vi "Simple Solenoid.vi"() -> ()   [LabVIEW 2025]
doc: "Simple Solenoid Example\n\nThis example shows how to set the value of a Solenoid Channel.\n\nIt works with the PCM (Pneumatic Control Module) communicating with the roboRIO over CAN bus. The PCM must also be supplied with 12V DC from the PDP (Power Distribution Panel).\n\nThe Compressor, Pressure Switch, and Solenoid are all wired to the PCM \n\nThis example expects a USB cable connected from your development PC to the Type B USB Jack (next to the power input) on the roboRIO.\n\nThis example expects the Driver Station to be running."
uses:
  <vilib>/Rock Robotics/WPI/Solenoid/WPI_SolenoidChannel.ctl
  <vilib>/Rock Robotics/WPI/Solenoid/WPI_SolenoidValue.ctl
  <vilib>/Rock Robotics/WPI/Solenoid/WPI_SolenoidOpenSingle.vi
  <vilib>/Rock Robotics/WPI/Solenoid/WPI_SolenoidSetEnum.vi
panel:
  in  "Select a PD device by clicking on the image below":u16(ring) items=["CTRE Pneumatic Module", "REV Pneumatics Hub"]
  in  "Solenoid Channel":T1
  in  "Value to Write":bool
  in  "stop":bool
  # "Wiring Diagram"
  # "Set this input before running."
  # "This can be set while running."
  # "On"
  # "Off"
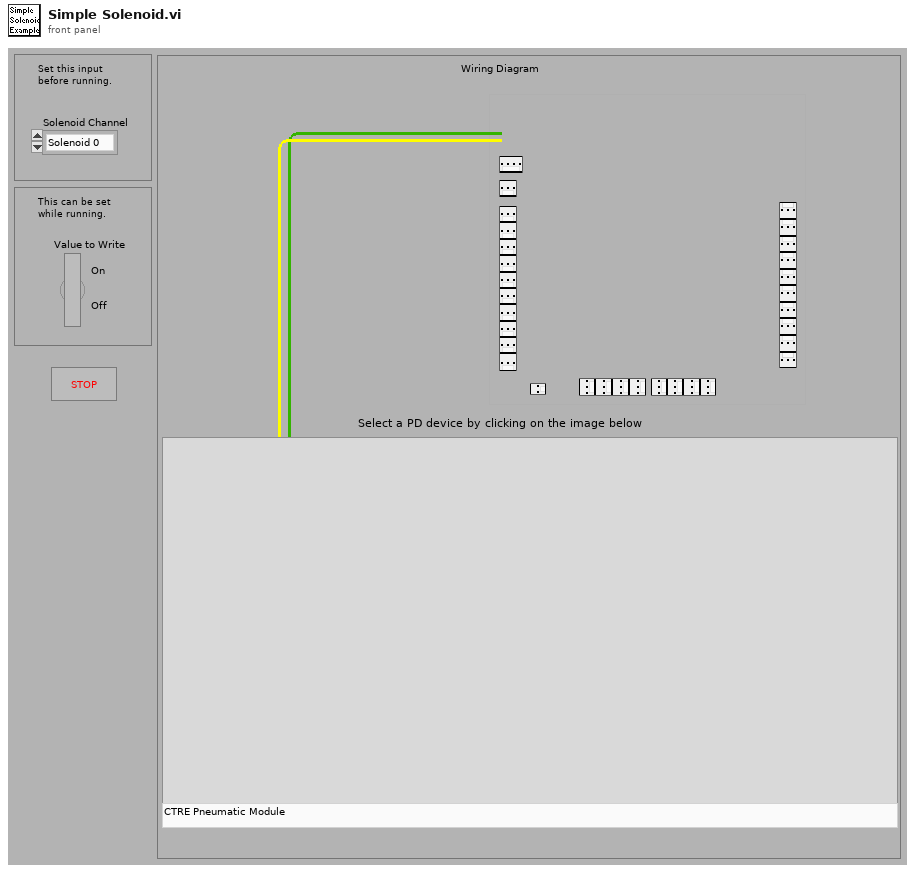
[diagram p1: front panel]
types:
  T1 = typedef "WPI_SolenoidChannel.ctl" = enum8{"Solenoid 0", "Solenoid 1", "Solenoid 2", "Solenoid 3", "Solenoid 4", "Solenoid 5", "Solenoid 6", "Solenoid 7", "Solenoid 8", "Solenoid 9", "Solenoid 10", "Solenoid 11", "Solenoid 12", "Solenoid 13", "Solenoid 14", "Solenoid 15", "Invalid"}
  T2 = typedef "WPI_SolenoidDevRef.ctl" = cluster{"DevStatus":errorcluster, "Pneumatics Control Module":u8, "Forward Solenoid Channel":T1, "Reverse Solenoid Channel":T1}
  T3 = typedef "WPI_SolenoidValue.ctl" = enum16{"Off", "On", "Forward", "Reverse"}
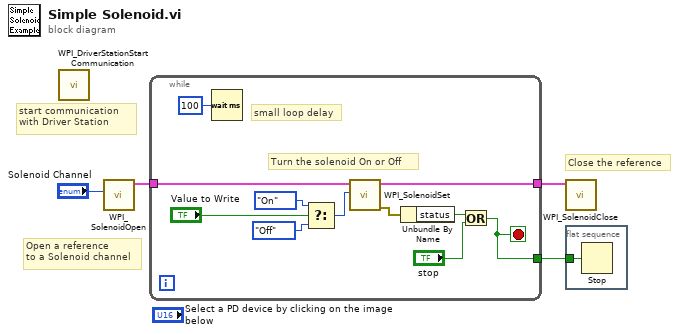
[diagram p0: block diagram]
diagram:
  # "start communication with Driver Station"
  # "Close the reference"
  # "Open a reference \nto a Solenoid channel"
  n1 = call <vilib>:"WPI_DriverStationStart Communication.vi"() -> ()  [unwired: 3 in, 9 out]
  n2 = call-poly <vilib>:"WPI_SolenoidOpen.vi"("Solenoid Channel"="Solenoid Channel") -> ("SolenoidDevRef"=w4:T2)  [unwired: 2 in, 8 out]
  n3 = while {
    tunnel: w4 -> [w14]
    tunnel: [w13] -> w3
    tunnel: [w9] -> w1
    stop <- w9 stop-if-true
    # "small loop delay"
    # "Turn the solenoid On or Off"
    n4 = Wait (ms)(milliseconds to wait=u32 100) -> ()  [unwired: 1 out]
    n5 = Select(t=WPI_SolenoidValue."On" ("Value"), s="Value to Write", f=WPI_SolenoidValue."Off" ("Value")) -> (s? t:f=w5:T3)
    n6 = call-poly <vilib>:"WPI_SolenoidSet.vi"("Value"=w5, "SolenoidDevRef"=w14) -> ("error out"=w12:errorcluster, "SolenoidDevRef"=w13:T2)  [unwired: 1 in, 7 out]
    n7 = Unbundle By Name(w12) -> ("status"=w11:bool)
    n8 = Or(x=w11, y="stop") -> (x .or. y?=w9:bool)
  }
  n9 = call <vilib>:"WPI_SolenoidClose.vi"("SolenoidDevRef"=w3) -> ()  [unwired: 1 in, 10 out]
  n10 = flat-sequence {
    tunnel: w1 -> [w16]
    frame #0 {
      n11 = Stop(stop? (T)=w16) -> ()
    }
  }
